vi "ChangeInheritance.vi"(0 "ClassWriterGOOP300 in":refnum<class "ClassWriterNative.lvclass">, 1 "LvClass":refnum<vi>, 2 "NewBaseClass(Empty=ConvertClassToBaseClass)":path=path "C:/Documents and Settings/Micke/Skrivbord/My Computer/B_class/B.lvclass", 5 "error in (no error)":errorcluster) -> (14 "ClassWriterGOOP300 out":refnum<class "ClassWriterNative.lvclass">, 19 "error out":errorcluster)   [LabVIEW 2020, in "ClassWriterNative.lvclass"]
uses:
  <resource>/Framework/Providers/Open_GDS/ClassProviders/Provider_LvNativeClass/ClassWriterNative_class/ClassWriterNative.lvclass
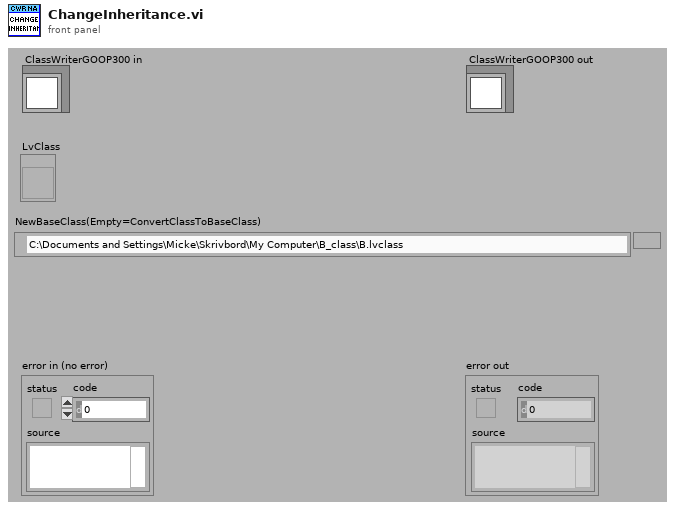
[diagram p1: front panel]
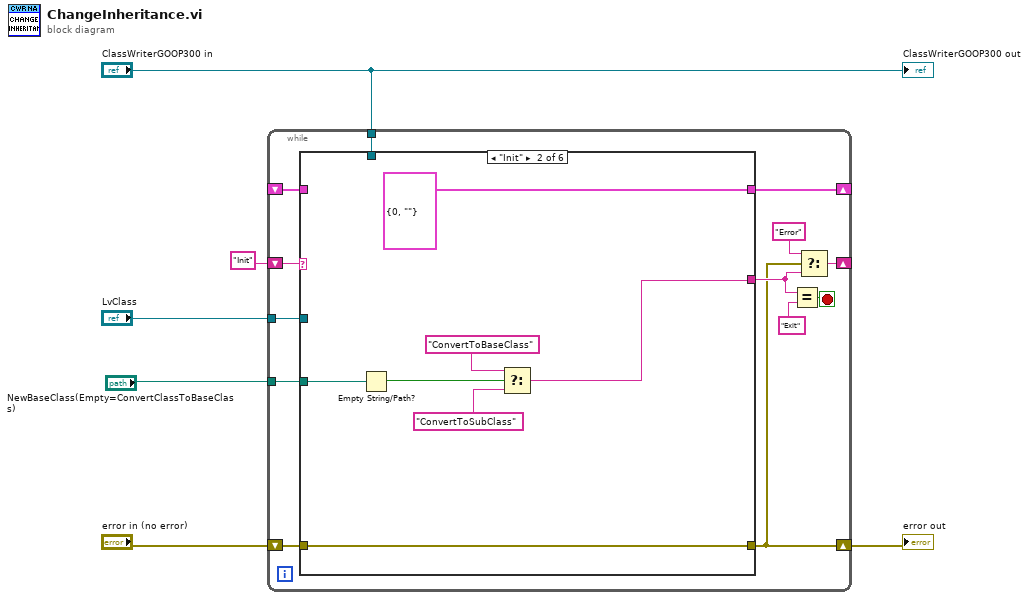
[diagram p0: block diagram]
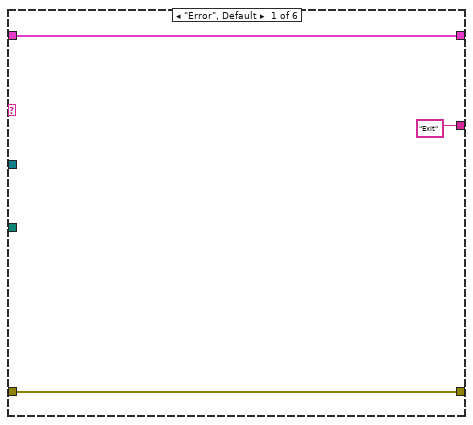
[diagram p2: hidden frame]
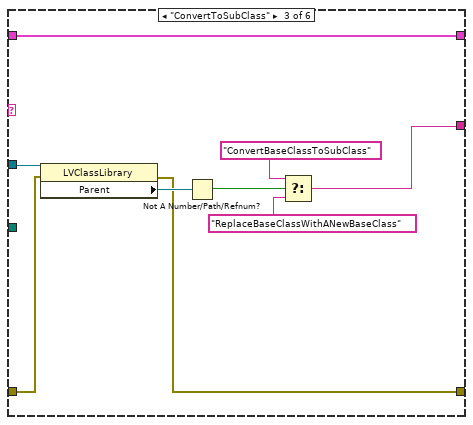
[diagram p3: hidden frame]
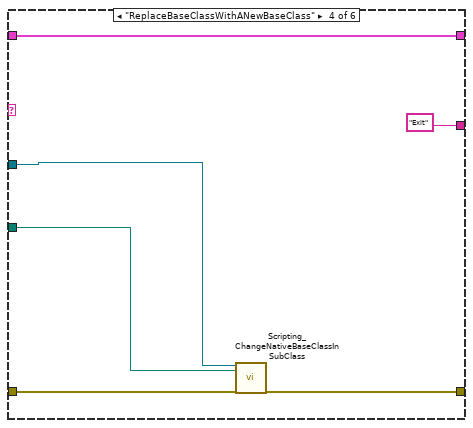
[diagram p4: hidden frame]
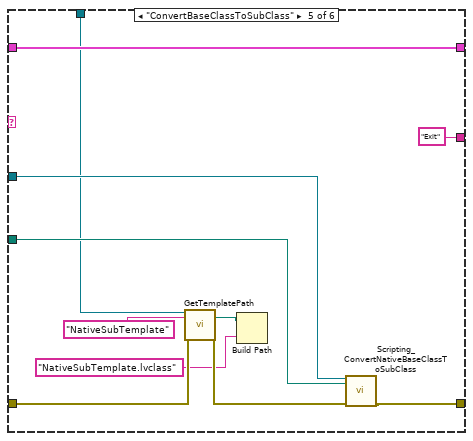
[diagram p5: hidden frame]
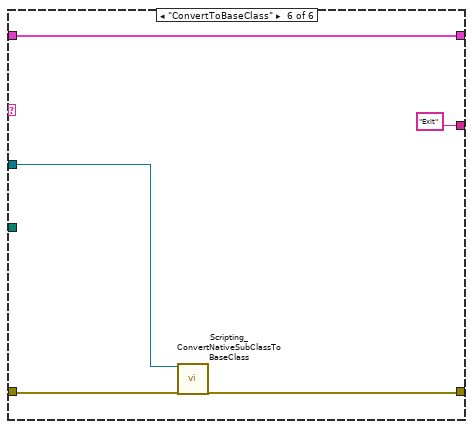
[diagram p6: hidden frame]
diagram:
  n1 = while {
    shift-right: [w13] -> w4
    shift-left: "error in (no error)" -> [w19]
    shift-right: [w17] -> _
    shift-left: "Init" -> [w18]
    shift-right: [w12] -> _
    shift-left: _ -> [w11]
    tunnel: "NewBaseClass(Empty=ConvertClassToBaseClass)" -> [w10]
    tunnel: "LvClass" -> [w9]
    tunnel: "ClassWriterGOOP300 in" -> [w7]
    stop <- w16 stop-if-true
    n2 = case shown="\"Init\"" w18 {
      tunnel: w19 -> [w22 w29 w37 w42 w51 w58]
      tunnel: [w22 w29 w32 w41 w55 w56] -> w13
      tunnel: ["Exit" w24 w33 "Exit" "Exit" "Exit"] -> w14
      tunnel: [w20 cluster{"Counter":i32, "Text":string} {"Counter"=0, "Text"=""} w30 w44 w46 w60] -> w12
      tunnel: w11 -> [w20 _ w30 w44 w46 w60]
      tunnel: w10 -> [_ w27 _ w39 w53 _]
      tunnel: w9 -> [_ _ w38 w40 w54 w57]
      tunnel: w7 -> [_ _ _ _ w45 _]
      frame "Error", Default {
      }
      frame "Init" {
        n3 = Empty String/Path?(string/path=w27) -> (empty?=w26:bool)
        n4 = Select(t="ConvertToBaseClass", s=w26, f="ConvertToSubClass") -> (s? t:f=w24:string)
      }
      frame "ConvertToSubClass" {
        n5 = property class="LVClassLibrary"(reference=w38, error in=w37) -> (error out=w32:errorcluster, "Parent"=w36:refnum<vi>)  [unwired: 1 out]
        n6 = Not A Number/Path/Refnum?(number/path/refnum=w36) -> (NaN/Path/Refnum?=w35:bool)
        n7 = Select(t="ConvertBaseClassToSubClass", s=w35, f="ReplaceBaseClassWithANewBaseClass") -> (s? t:f=w33:string)
      }
      frame "ReplaceBaseClassWithANewBaseClass" {
        n8 = call <resource>:"Scripting_ChangeNativeBaseClassInSubClass.vi"("SubClass"=w40, "NewBaseClass"=w39, "error in (no error)"=w42) -> ("error out"=w41:errorcluster)  [unwired: 16 in]
      }
      frame "ConvertBaseClassToSubClass" {
        n9 = call-dynamic "GetTemplatePath.vi"("reference in"=w45, "ClassTemplateSubDirectory"="NativeSubTemplate", "error in (no error)"=w51) -> ("FolderPathOut"=w49:path, "error out"=w50:errorcluster)  [unwired: 12 in, 3 out]
        n10 = Build Path(base path=w49, name or relative path="NativeSubTemplate.lvclass") -> ()  [unwired: 1 out]
        n11 = call <resource>:"Scripting_ConvertNativeBaseClassToSubClass.vi"("BaseClass"=w54, "NewBaseClass"=w53, "error in (no error)"=w50) -> ("error out"=w55:errorcluster)  [unwired: 16 in]
      }
      frame "ConvertToBaseClass" {
        n12 = call <resource>:"Scripting_ConvertNativeSubClassToBaseClass.vi"("SubClass"=w57, "error in (no error)"=w58) -> ("error out"=w56:errorcluster)  [unwired: 17 in]
      }
    }
    n13 = Equal?(x=w14, y="Exit") -> (x = y?=w16:bool)
    n14 = Select(t="Error", s=w13, f=w14) -> (s? t:f=w17:string)
  }
  "error out" <- w4
  "ClassWriterGOOP300 out" <- "ClassWriterGOOP300 in"
